vi "UART Close Device.vi"(10 "DevIndex":i32, 11 "DevType":i32) -> (3 "function return":i32)   [LabVIEW 2010, in "ControlUART.lvlib"]
doc: "int WINAPI UART_CloseDevice(int DevType,int DevIndex);"
uses:
  ControlUART.lvlib
  ControlUART/Ginkgo_Driver.dll
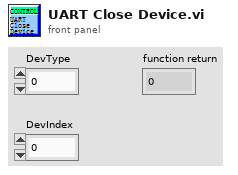
[diagram p1: front panel]
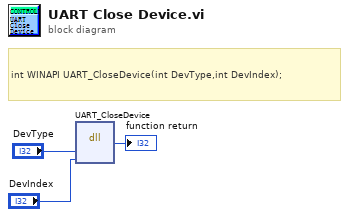
[diagram p0: block diagram]
diagram:
  # "int WINAPI UART_CloseDevice(int DevType,int DevIndex);"
  n1 = dll-call lib="E:/Project/vt_ginkgo/truck/Ginkgo Driver/vs2010/Ginkgo_USB-I2C&SPI&CAN_API_v2.0.3.3/lib/labview_32bit/ControlUART/Ginkgo_Driver.*" fn="UART_CloseDevice"("DevType"="DevType", "DevIndex"="DevIndex") -> (→"function return":i32)  [unwired: 5 in, 2 out]
